vi "Finding Specific Folder in Projects.vi"(7 "Interation Counts":i32=50, 10 "Target":string="Support Folder", 11 "Start Path":path) -> (2 "Find":bool, 3 "Path Out":path)   [LabVIEW 2024]
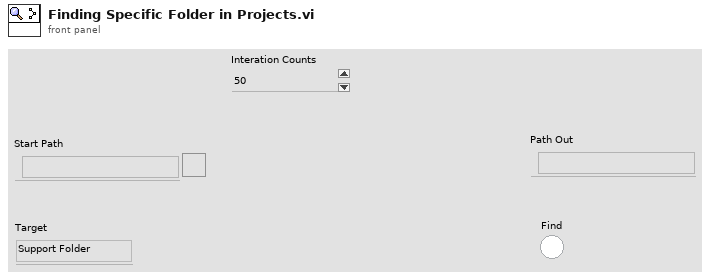
[diagram p1: front panel]
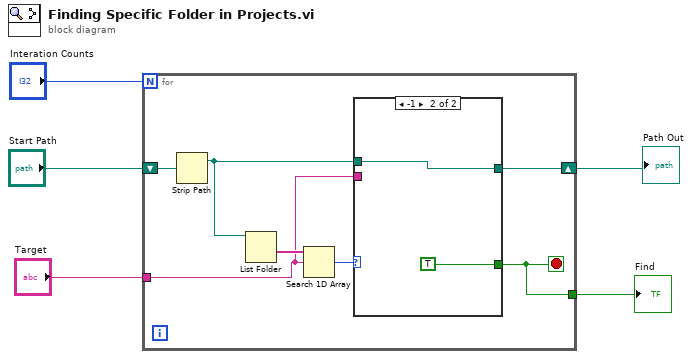
[diagram p0: block diagram]
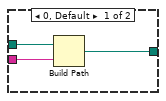
[diagram p2: hidden frame]
diagram:
  n1 = for {
    N: "Interation Counts" -> [_]
    shift-right: [w8] -> w3
    shift-left: "Start Path" -> [w12]
    tunnel: "Target" -> [w7]
    tunnel: [w6] -> w1
    stop <- w6 stop-if-true
    n2 = Strip Path(path=w12) -> (stripped path=w9:path)  [unwired: 1 out]
    n3 = List Folder(path=w9) -> (folder names=w11:string[])  [unwired: 3 in, 3 out]
    n4 = Search 1D Array(1D array=w11, element=w7) -> (index of element=w10:i32)  [unwired: 1 in]
    n5 = case shown="-1" w10 {
      tunnel: w9 -> [w15 w17]
      tunnel: [w13 w17] -> w8
      tunnel: w7 -> [w14 _]
      tunnel: [_ TRUE] -> w6
      frame 0, Default {
        n6 = Build Path(base path=w15, name or relative path=w14) -> (appended path=w13:path)
      }
      frame -1 {
      }
    }
  }
  "Path Out" <- w3
  "Find" <- w1
